vi "sub_alarm-led.vi"(7 "alarm":T1(ring), 8 "error in":errorcluster, 11 "onoff":bool) -> (0 "error out":errorcluster)   [LabVIEW 2019]
uses:
  Devices/NI Board/cDAQ-9476 DO/cnt_Relay.ctl
  Devices/NI Board/cDAQ-9476 DO/cnt_do.ctl
  Global 1.vi
  UI.ctl
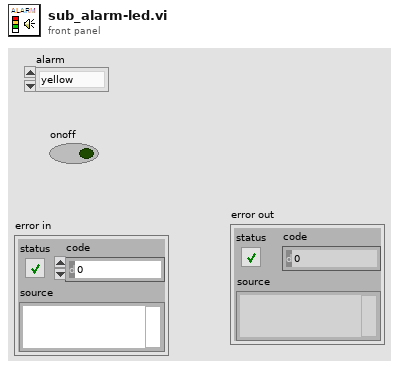
[diagram p1: front panel]
types:
  T1 = enum16{"yellow", "red", "green", "buzz1", "buzz2"}
  T2 = typedef "cnt_Relay.ctl" = enum32{"R_Load", "R_out1", "R_out2", "R_out3", "R_out4", "R_out5", "R_out6", "R8", "R9", "R10", "R11", "R12", "R13", "R14", "R15", "R16", "R_in1", "R_in2", "R_in3", "R_in4", "R_in5", "R_in6", "R23", "R24", "R25", "R26", "R27", "R_red", "R_yellow", "R_green", "R_buz", "R_purple"}
  T3 = typedef "cnt_do.ctl" = enum16{"open", "initial", "update", "run", "close"}
  T4 = typedef "UI.ctl" = enum16{"Alarm yellow", "DL950 graph show", "DL950 graph clear", "AO value", "AO blink onoff", "Discharge relay", "Input Power", "Outpower", "Relay in1", "Relay in2", "Relay in3", "Relay in4", "Relay in5", "Relay in6", "Relay out1", "Relay out2", "Relay out3", "Relay out4", "Relay out5", "Relay out6", "Relay all off"}
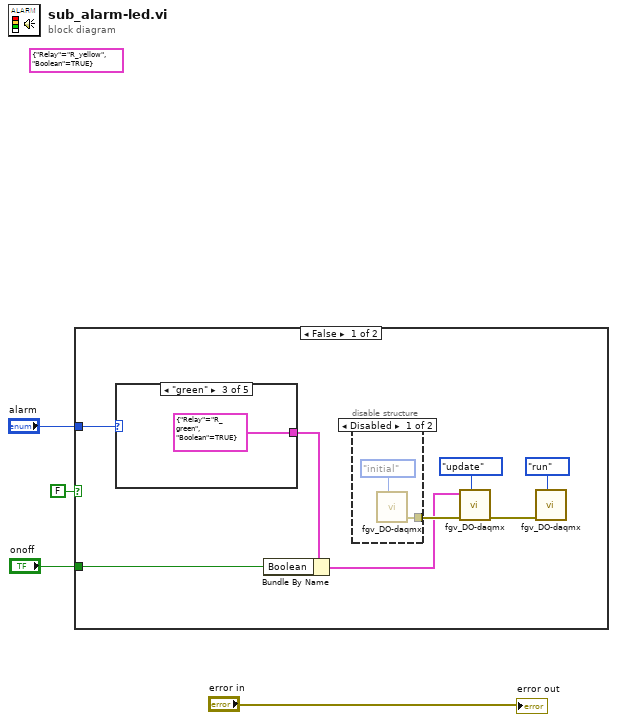
[diagram p0: block diagram]
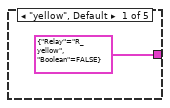
[diagram p3: hidden frame]
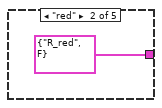
[diagram p4: hidden frame]
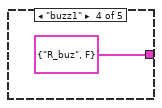
[diagram p5: hidden frame]
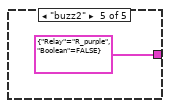
[diagram p6: hidden frame]
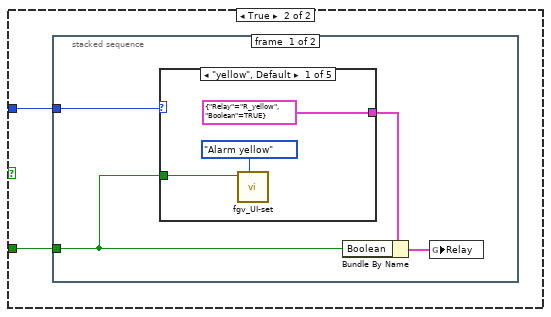
[diagram p7: hidden frame]
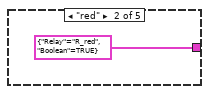
[diagram p8: hidden frame]
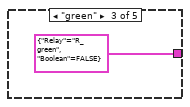
[diagram p9: hidden frame]
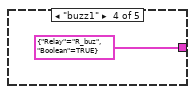
[diagram p10: hidden frame]
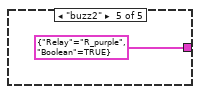
[diagram p11: hidden frame]
diagram:
  (unwired) cluster{"Relay":T2, "Boolean":bool} {"Relay"=enum."R_yellow", "Boolean"=TRUE} ("Relay")
  n1 = case shown="False" FALSE {
    tunnel: "alarm" -> [w8 w21]
    tunnel: "onoff" -> [w6 w20]
    frame False {
      n2 = case shown="\"green\"" w8 {
        tunnel: [cluster{"Relay":T2, "Boolean":bool} {"Relay"=enum."R_yellow", "Boolean"=FALSE} ("Relay") cluster{"Relay":T2, "Boolean":bool} {"Relay"=enum."R_red", "Boolean"=FALSE} ("Relay") cluster{"Relay":T2, "Boolean":bool} {"Relay"=enum."R_green", "Boolean"=TRUE} ("Relay") cluster{"Relay":T2, "Boolean":bool} {"Relay"=enum."R_buz", "Boolean"=FALSE} ("Relay") cluster{"Relay":T2, "Boolean":bool} {"Relay"=enum."R_purple", "Boolean"=FALSE} ("Relay")] -> w7
        frame "yellow", Default {
        }
        frame "red" {
        }
        frame "green" {
        }
        frame "buzz1" {
        }
        frame "buzz2" {
        }
      }
      n3 = Bundle By Name(cluster=w7, "Boolean"=w6) -> (w5:cluster{"Relay":T2, "Boolean":bool})
      n4 = disable-structure shown="Disabled" {
        disable-tunnel: [w13 _] -> w11
        frame Disabled {
          n5 = call "fgv_DO-daqmx.vi"("cnt"=cnt_do."initial") -> ("error out"=w13:errorcluster)  [unwired: 10 in]
        }
        frame Enabled {
        }
      }
      n6 = call "fgv_DO-daqmx.vi"("cnt"=cnt_do."update", "error in"=w11, "Relay"=w5) -> ("error out"=w9:errorcluster)  [unwired: 8 in]
      n7 = call "fgv_DO-daqmx.vi"("cnt"=cnt_do."run", "error in"=w9) -> ()  [unwired: 9 in, 1 out]
    }
    frame True {
      n8 = stacked-sequence {
        tunnel: w21 -> [w23 _]
        tunnel: w20 -> [w22 _]
        frame #0 {
          n9 = case shown="\"yellow\", Default" w23 {
            tunnel: [cluster{"Relay":T2, "Boolean":bool} {"Relay"=enum."R_yellow", "Boolean"=TRUE} ("Relay") cluster{"Relay":T2, "Boolean":bool} {"Relay"=enum."R_red", "Boolean"=TRUE} ("Relay") cluster{"Relay":T2, "Boolean":bool} {"Relay"=enum."R_green", "Boolean"=FALSE} ("Relay") cluster{"Relay":T2, "Boolean":bool} {"Relay"=enum."R_buz", "Boolean"=TRUE} ("Relay") cluster{"Relay":T2, "Boolean":bool} {"Relay"=enum."R_purple", "Boolean"=TRUE} ("Relay")] -> w24
            tunnel: w22 -> [w26 _ _ _ _]
            frame "yellow", Default {
              n10 = call "fgv_UI-set.vi"("cmd"=UI."Alarm yellow", "onoff"=w26) -> ()  [unwired: 9 in, 1 out]
            }
            frame "red" {
            }
            frame "green" {
            }
            frame "buzz1" {
            }
            frame "buzz2" {
            }
          }
          n11 = Bundle By Name(cluster=w24, "Boolean"=w22) -> (w25:cluster{"Relay":T2, "Boolean":bool})
          n12 = global write "Global 1.vi" "Relay"(w25) -> ()
        }
        frame #1 {
        }
      }
    }
  }
  "error out" <- "error in"
